vi "FPGA_Rates_subVI.vi"(9 "Fs In (Hz)":dbl=100000.0 format="%#_6p", 10 "Fs Out (Hz)":dbl=40000.0 format="%#_6p", 11 "Chirp Len (ms)":dbl) -> (1 "# Output Samples":i16, 2 "Input Ticks (ticks/S)":u32, 3 "Output Ticks (ticks/S)":u32, 4 "Chirp Len (ms)":dbl)   [LabVIEW 2017]
doc: "Initializes rates for FPGA input and output based on the 40 MHZ clock."
uses:
  <vilib>/rvi/Analysis/host/Private/Sample Rate To Loop Time (ticks).vi
  <vilib>/rvi/Analysis/host/Public/NI_FpgaMspHost.lvlib
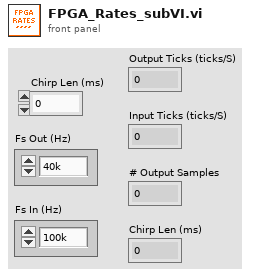
[diagram p1: front panel]
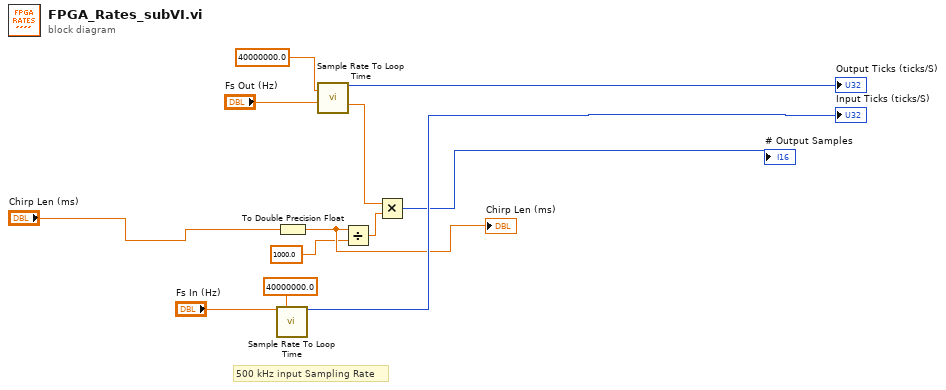
[diagram p0: block diagram]
diagram:
  # "500 kHz input Sampling Rate"
  n1 = call-poly <vilib>:"Sample Rate To Loop Time.vi"("sample rate (S/s)"="Fs In (Hz)", "FPGA clock rate (Hz)"=40000000.0) -> ("count (ticks/S)"=→"Input Ticks (ticks/S)":u32)  [unwired: 11 in, 2 out]
  n2 = To Double Precision Float(number="Chirp Len (ms)") -> (double precision float=w9:dbl)
  "Chirp Len (ms)" <- w9
  n3 = call-poly <vilib>:"Sample Rate To Loop Time.vi"("sample rate (S/s)"="Fs Out (Hz)", "FPGA clock rate (Hz)"=40000000.0) -> ("count (ticks/S)"=→"Output Ticks (ticks/S)":u32, "actual sample rate (S/s)"=w7:dbl)  [unwired: 11 in, 1 out]
  n4 = Divide(x=w9, y=1000.0) -> (x/y=w8:dbl)
  n5 = Multiply(x=w7, y=w8) -> (x*y=→"# Output Samples":i16)
